vi "Q Driver 1.vi"(8 "error in":errorcluster, 9 "Enum":T2, 10 "EnQ/Enstack":T1[](array[typedef]), 11 "name":string) -> (0 "error out":errorcluster, 1 "# elements in queue":i32, 2 "DQ ele":T1)   [LabVIEW 2020]
uses:
  Controller/Queue Controller.ctl
  Controller/Main Controller.ctl
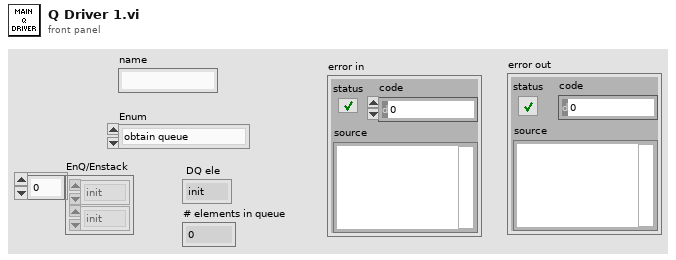
[diagram p1: front panel]
types:
  T1 = typedef "Main Controller.ctl" = enum16{"init", "poll", "read file", "update md cluster ", "precheck", "display", "Calculate", "timer", "update file", "reset", "error", "exit"}
  T2 = typedef "Queue Controller.ctl" = enum16{"obtain queue", "enqueue", "dequeue", "enstack", "release que", "get queue stat"}
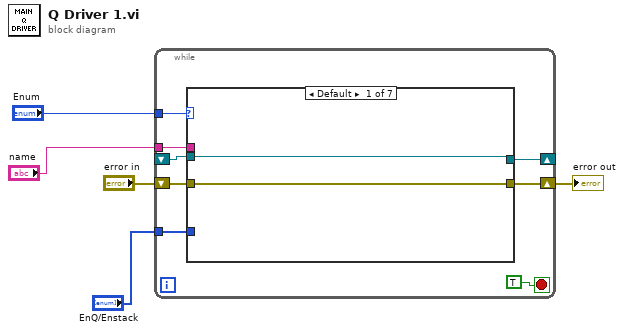
[diagram p0: block diagram]
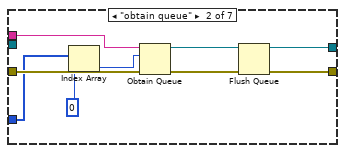
[diagram p2: hidden frame]
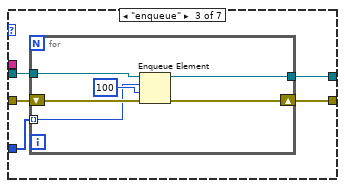
[diagram p3: hidden frame]
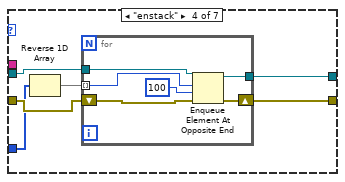
[diagram p4: hidden frame]
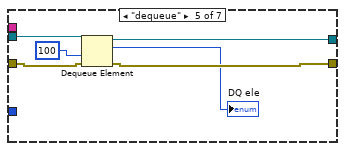
[diagram p5: hidden frame]
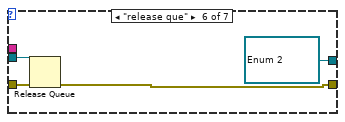
[diagram p6: hidden frame]
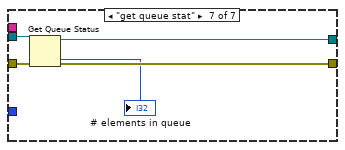
[diagram p7: hidden frame]
diagram:
  n1 = while {
    shift-right: [w11] -> w4
    shift-left: "error in" -> [w12]
    tunnel: "Enum" -> [w10]
    tunnel: "EnQ/Enstack" -> [w9]
    shift-right: [w8] -> _
    shift-left: _ -> [w7]
    tunnel: "name" -> [w6]
    stop <- TRUE stop-if-true
    n2 = case shown="Default" w10 {
      tunnel: w12 -> [w15 w22 w29 w41 w53 w57 w62]
      tunnel: [w15 w21 w28 w40 w52 w56 w61] -> w11
      tunnel: w9 -> [_ w20 w27 w39 _ _ _]
      tunnel: [w14 w17 w26 w36 w49 w54 w59] -> w8
      tunnel: w7 -> [w14 _ w25 w37 w50 w55 w60]
      tunnel: w6 -> [_ w16 _ _ _ _ _]
      frame Default {
      }
      frame "obtain queue" {
        n3 = Index Array(array=w20, index=0) -> (element=w18:T1)
        n4 = Obtain Queue(name (unnamed)=w16, element data type=w18, error in (no error)=w22) -> (queue out=w23:refnum<queue>, error out=w24:errorcluster)  [unwired: 2 in, 1 out]
        n5 = Flush Queue(queue=w23, error in (no error)=w24) -> (queue out=w17:refnum<queue>, error out=w21:errorcluster)  [unwired: 1 out]
      }
      frame "enqueue" {
        n6 = for {
          tunnel: [w33] -> w26
          tunnel: w27 -> [w30] mode=indexing
          shift-right: [w34] -> w28
          shift-left: w29 -> [w35]
          tunnel: w25 -> [w31]
          n7 = Enqueue Element(queue=w31, element=w30, timeout in ms (-1)=100, error in (no error)=w35) -> (queue out=w33:refnum<queue>, error out=w34:errorcluster)  [unwired: 1 out]
        }
      }
      frame "enstack" {
        n8 = Reverse 1D Array(array=w39) -> (reversed array=w38:T1[])
        n9 = for {
          tunnel: [w45] -> w36
          tunnel: w38 -> [w42] mode=indexing
          shift-right: [w46] -> w40
          shift-left: w41 -> [w47]
          tunnel: w37 -> [w43]
          n10 = Enqueue Element At Opposite End(queue=w43, element=w42, timeout in ms (-1)=100, error in (no error)=w47) -> (queue out=w45:refnum<queue>, error out=w46:errorcluster)  [unwired: 1 out]
        }
      }
      frame "dequeue" {
        n11 = Dequeue Element(queue=w50, timeout in ms (-1)=100, error in (no error)=w53) -> (queue out=w49:refnum<queue>, element=→"DQ ele":T1, error out=w52:errorcluster)  [unwired: 1 out]
      }
      frame "release que" {
        w54 = refnum<queue> refnum items=["init", "poll", "read file", "update md cluster ", "precheck", "display", "Calculate", "timer", "update file", "reset", "error", "exit"] ("queue out")
        n12 = Release Queue(queue=w55, error in (no error)=w57) -> (error out=w56:errorcluster)  [unwired: 1 in, 2 out]
      }
      frame "get queue stat" {
        n13 = Get Queue Status(queue=w60, error in (no error)=w62) -> (queue out=w59:refnum<queue>, error out=w61:errorcluster, # elements in queue=→"# elements in queue":i32)  [unwired: 1 in, 5 out]
      }
    }
  }
  "error out" <- w4
